vi "CommandList.vi"() -> (3 "Array":string[](array[string]))   [LabVIEW 2016]
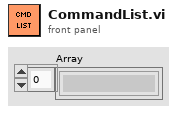
[diagram p1: front panel]
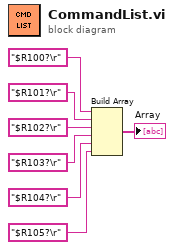
[diagram p0: block diagram]
diagram:
  n1 = Build Array("$R100?\r" ("string to write"), "$R101?\r" ("string to write"), "$R102?\r" ("string to write"), "$R103?\r" ("string to write"), "$R104?\r" ("string to write"), "$R105?\r" ("string to write")) -> (→"Array":string[])
